vi "Get shift date time range.vi"(0 "time stamp":timestamp, 11 "error in (no error)":errorcluster) -> (2 "1st shift 1st half start":string, 3 "1st shift 1st half end":string, 4 "2nd shift 1st half start":string, 6 "2nd shift 1st half end":string, 8 "2nd shift 2nd half start":string, 10 "2nd shift 2nd half end":string, 13 "1st shift 2nd half start":string, 14 "1st shift 2nd half end":string, 15 "error out":errorcluster)   [LabVIEW 2013]
panel:
  out "Next day year":u32
  out "Next day date":u32
  out "Next day month":u32
  in  "Days in month":u32[](array[numeric])=[31, 28, 31, 30, 31, 30, 31, 31, 30, 31, 30, 31]
  out "Timestamp from Number of Seconds":timestamp
  out "year":string
  out "Day":string
  out "Month":string
  out "date/time string":string
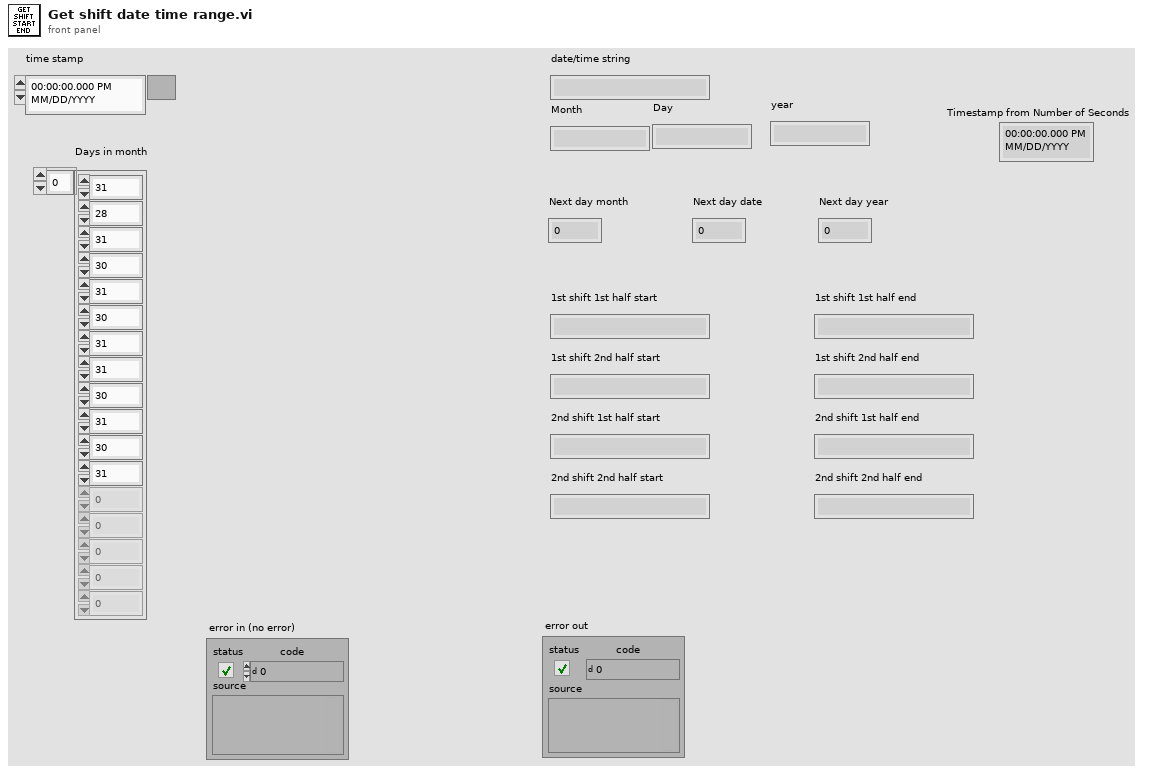
[diagram p1: front panel]
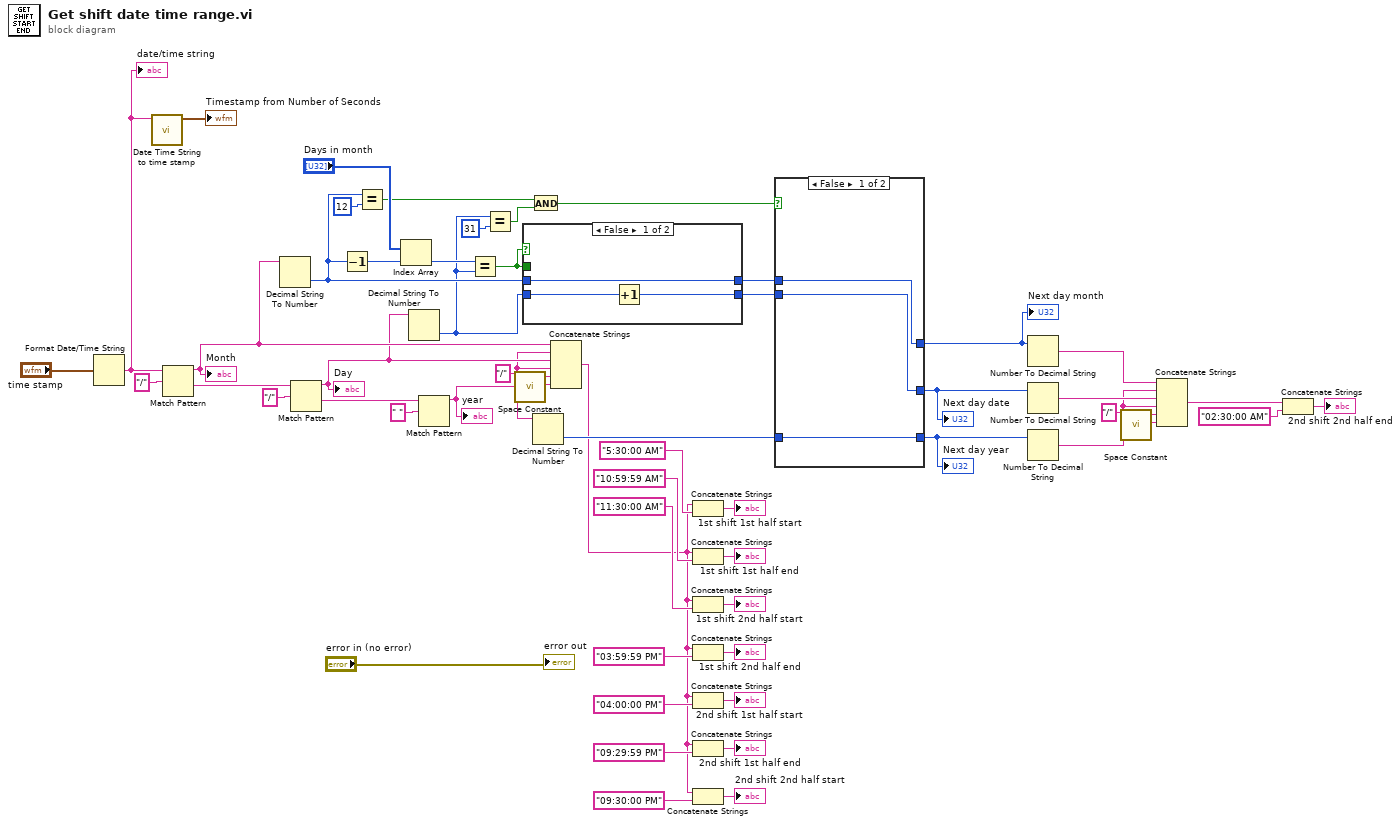
[diagram p0: block diagram]
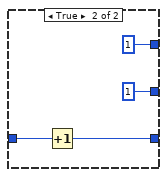
[diagram p2: hidden frame]
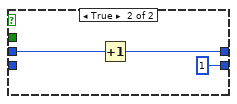
[diagram p3: hidden frame]
diagram:
  w11 = "/" ("string")
  w29 = "/" ("string")
  n1 = Format Date/Time String(seconds (now)="time stamp") -> (date/time string=w48:string)  [unwired: 2 in]
  "date/time string" <- w48
  n2 = call "Date Time String to time stamp.vi"("Sample Date Time String"=w48) -> ("Timestamp from Number of Seconds"=→"Timestamp from Number of Seconds":timestamp)  [unwired: 9 in, 1 out]
  n3 = Match Pattern(string=w48, regular expression="/") -> (before substring=w32:string, after substring=w51:string)  [unwired: 1 in, 2 out]
  "Month" <- w32
  n4 = Decimal String To Number(string=w32) -> (number=w43:i32)  [unwired: 2 in, 1 out]
  n5 = Match Pattern(string=w51, regular expression="/") -> (before substring=w31:string, after substring=w49:string)  [unwired: 1 in, 2 out]
  "Day" <- w31
  n6 = Decrement(x=w43) -> (x-1=w46:i32)
  n7 = Equal?(x=w43, y=12) -> (x = y?=w38:bool)
  n8 = Index Array(array="Days in month", index=w46) -> (element=w41:u32)
  n9 = Decimal String To Number(string=w31) -> (number=w40:i32)  [unwired: 2 in, 1 out]
  n10 = Match Pattern(string=w49, regular expression=" ") -> (before substring=w30:string)  [unwired: 1 in, 3 out]
  "year" <- w30
  n11 = Equal?(x=w41, y=w40) -> (x = y?=w44:bool)
  n12 = Equal?(x=w40, y=31) -> (x = y?=w37:bool)
  n13 = call <vilib>:"Space Constant.vi"() -> ("String"=w28:string)
  n14 = case shown="False" w44 {
    tunnel: w44 -> [_ _]
    tunnel: w40 -> [w55 _]
    tunnel: [w56 1] -> w33
    tunnel: w43 -> [w57 w59]
    tunnel: [w57 w58] -> w34
    frame False {
      n15 = Increment(x=w55) -> (x+1=w56:i32)
    }
    frame True {
      n16 = Increment(x=w59) -> (x+1=w58:i32)
    }
  }
  n17 = And(x=w38, y=w37) -> (x .and. y?=w36:bool)
  n18 = Decimal String To Number(string=w30) -> (number=w35:i32)  [unwired: 2 in, 1 out]
  n19 = Concatenate Strings(w32, w29, w31, w29, w30, w28) -> (w5:string)
  n20 = Concatenate Strings(w5, "5:30:00 AM" ("string")) -> (→"1st shift 1st half start":string)
  n21 = Concatenate Strings(w5, "10:59:59 AM" ("string")) -> (→"1st shift 1st half end":string)
  n22 = Concatenate Strings(w5, "11:30:00 AM" ("string")) -> (→"1st shift 2nd half start":string)
  n23 = Concatenate Strings(w5, "03:59:59 PM" ("string")) -> (→"1st shift 2nd half end":string)
  n24 = Concatenate Strings(w5, "04:00:00 PM" ("string")) -> (→"2nd shift 1st half start":string)
  n25 = Concatenate Strings(w5, "09:29:59 PM" ("string")) -> (→"2nd shift 1st half end":string)
  n26 = Concatenate Strings(w5, "09:30:00 PM" ("string")) -> (→"2nd shift 2nd half start":string)
  n27 = case shown="False" w36 {
    tunnel: w35 -> [w63 w67]
    tunnel: [w63 w66] -> w14
    tunnel: [w62 1] -> w15
    tunnel: w34 -> [w62 _]
    tunnel: w33 -> [w61 _]
    tunnel: [w61 1] -> w16
    frame False {
    }
    frame True {
      n28 = Increment(x=w67) -> (x+1=w66:i32)
    }
  }
  "Next day month" <- w15
  "Next day date" <- w16
  "Next day year" <- w14
  n29 = Number To Decimal String(number=w15) -> (decimal integer string=w13:string)  [unwired: 1 in]
  n30 = Number To Decimal String(number=w16) -> (decimal integer string=w12:string)  [unwired: 1 in]
  n31 = Number To Decimal String(number=w14) -> (decimal integer string=w10:string)  [unwired: 1 in]
  n32 = call <vilib>:"Space Constant.vi"() -> ("String"=w9:string)
  n33 = Concatenate Strings(w13, w11, w12, w11, w10, w9) -> (w8:string)
  n34 = Concatenate Strings(w8, "02:30:00 AM" ("string")) -> (→"2nd shift 2nd half end":string)
  "error out" <- "error in (no error)"
